vi "macro_SwerveDriveKineNew4.vi"   [LabVIEW 2019, in "Trajectory_Library.lvlib"]
uses:
  Trajectory_Library.lvlib
types:
  T1 = typedef "Trajectory_Library.lvlib/TRANSLATION2D.ctl" = cluster{"X":dbl, "Y":dbl}
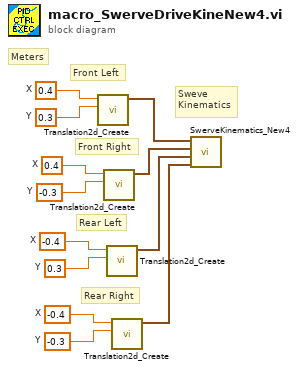
[diagram p0: block diagram]
diagram:
  w5 = -0.4  # X
  w6 = -0.3  # Y
  w7 = -0.4  # X
  w8 = 0.3  # Y
  w9 = 0.4  # X
  w10 = -0.3  # Y
  w11 = 0.4  # X
  w12 = 0.3  # Y
  # "Meters"
  # "Sweve\nKinematics"
  # "Rear Right"
  # "Rear Left"
  # "Front Right"
  # "Front Left"
  n1 = call "Translation2d_Create.vi"("Y"=w12, "X"=w11) -> ("TRANSLATION"=w4:T1)  [unwired: 9 in]
  n2 = call "Translation2d_Create.vi"("Y"=w10, "X"=w9) -> ("TRANSLATION"=w3:T1)  [unwired: 9 in]
  n3 = call "Translation2d_Create.vi"("Y"=w8, "X"=w7) -> ("TRANSLATION"=w2:T1)  [unwired: 9 in]
  n4 = call "Translation2d_Create.vi"("Y"=w6, "X"=w5) -> ("TRANSLATION"=w1:T1)  [unwired: 9 in]
  n5 = call "SwerveKinematics_New4.vi"("wheel 3"=w1, "wheel 2"=w2, "wheel 1"=w3, "wheel 0"=w4) -> ()  [unwired: 7 in, 1 out]
